vi "Test RoundTrip Nulls.vi"(8 "error in (no error)":errorcluster) -> (0 "error out":errorcluster)   [LabVIEW 2015]
uses:
  <vilib>/Utility/VariantDataType/Type.ctl
  src/Serializer/JSON Serializer/JSON Serializer.lvclass
  src/Deserializer/JSON Deserializer/JSON Deserializer.lvclass
  <vilib>/addons/_JKI Toolkits/Caraya/classes/Test/Test.lvclass
  <vilib>/addons/_JKI Toolkits/Caraya/classes/Assert/Assert.lvclass
  src/JKI JSON Serialization.lvlib
  <vilib>/Utility/VariantDataType/VariantType.lvlib
panel:
  out "Type Enum 2":T1
  out "Wrapped void variant input":cluster{"variant":variant}
  out "Wrapped void variant output":cluster{"variant":variant}
  out "I think this should be {}":string
  out "data":string
  out "Name 3":string
  out "Name":string
  out "output cluster":cluster{"variant container":variant}
  out "I think this should be {\"variant\":null}":string
  out "Type Enum":T1
  out "I think this should be {\"variant\":{}}":string
  out "I think this should be {\"variant\":{}}":string
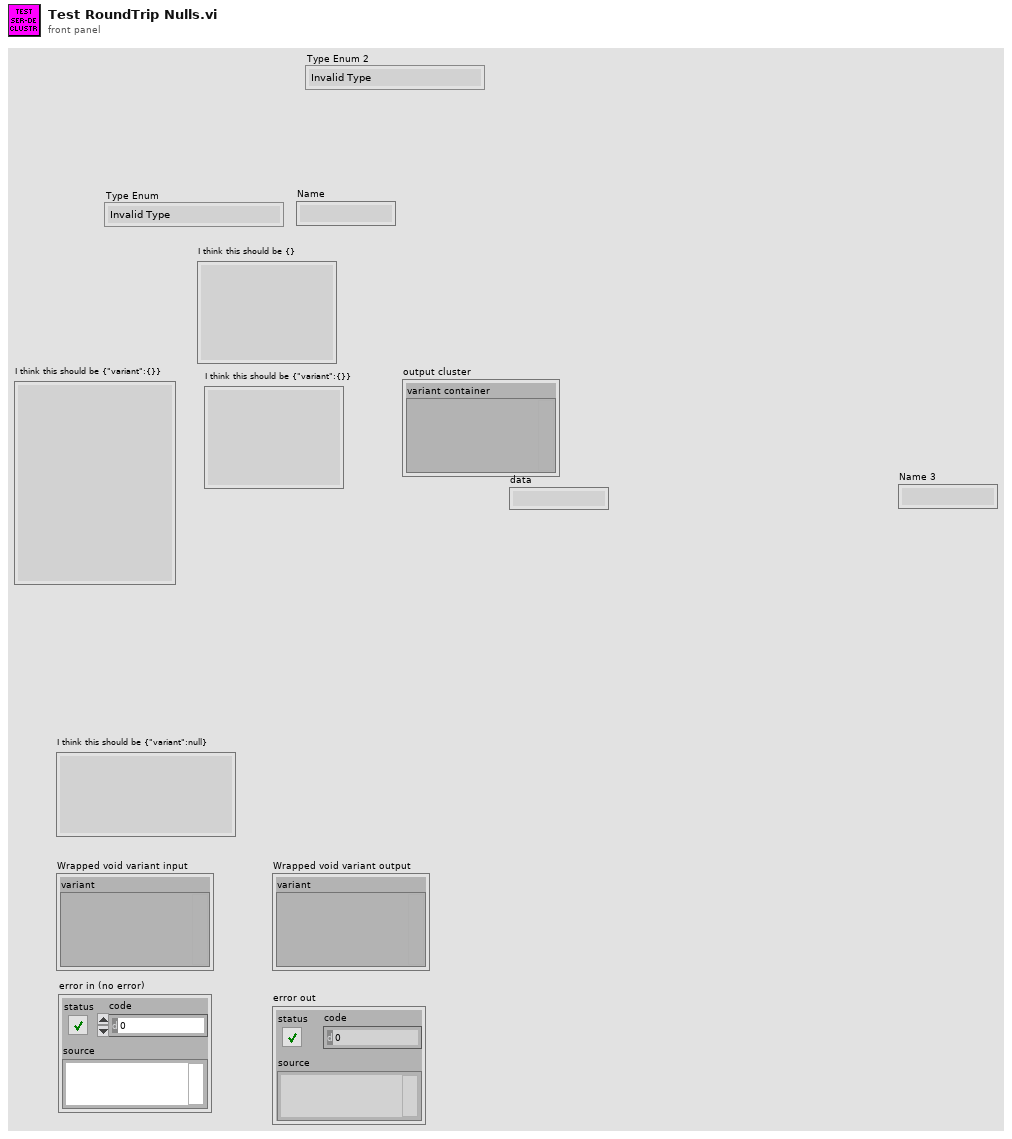
[diagram p1: front panel]
types:
  T1 = typedef "VariantType.lvlib/Type.ctl" = enum8{"Invalid Type", "Void", "I8", "I16", "I32", "I64", "U8", "U16", "U32", "U64", "Single Float", "Double Float", "Extended Float", "Single Complex", "Double Complex", "Extended Complex", "Enum U8", "Enum U16", "Enum U32", "Enum U64", "Single Float With Unit", "Double Float With Unit", "Extended Float With Unit", "Single Complex with Unit", "Double Complex with Unit", "Extended Complex with Unit", "Boolean", "String", "Path", "Picture", "Tag", "Array", "Cluster", "Variant", "LV Variant", "Waveform", "Timestamp", "Digital Waveform", "Digital Data", "ExpressData", "Refnum", "External Data", "VI", "Poly VI", "LabVIEW Class Instance", "Fixed Point"}
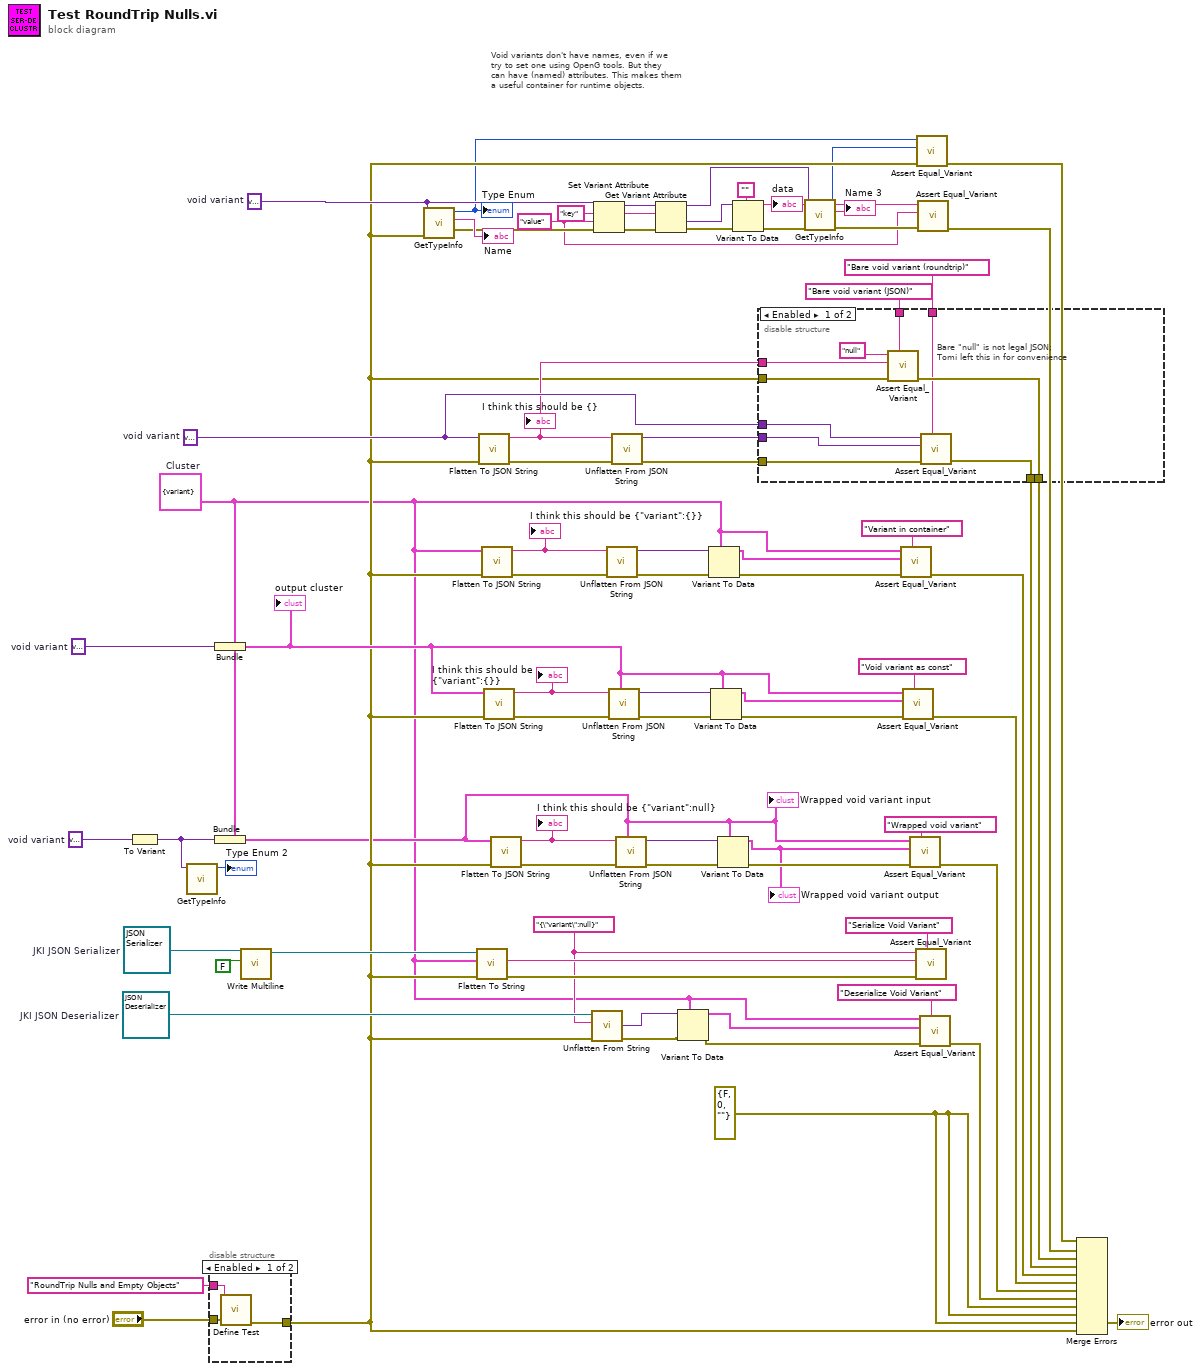
[diagram p0: block diagram]
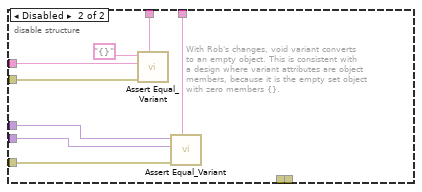
[diagram p2: hidden frame]
diagram:
  w7 = "{\"variant\":null}" ("String")
  w4 = cluster{"variant":variant} {"variant"=variant}  # Cluster
  w13 = "value" ("name")
  w34 = "key" ("name")
  w26 = variant  # void variant
  w39 = variant  # void variant
  w21 = variant  # void variant
  w54 = refnum<class "JSON Deserializer.lvclass"> refnum  # JKI JSON Deserializer
  w57 = refnum<class "JSON Serializer.lvclass"> refnum  # JKI JSON Serializer
  w3 = errorcluster {"status"=FALSE, "code"=0, "source"=""} ("error out")
  w38 = variant  # void variant
  # "Void variants don't have names, even if we\ntry to set one using OpenG tools. But they \ncan have (named) attributes. This makes them\na useful container for runtime objects."
  n1 = To Variant(anything=w39) -> (Variant=w2:variant)
  n2 = call <vilib>:"GetTypeInfo.vi"("Variant"=w2) -> ("Type Enum"=→"Type Enum 2":T1)  [unwired: 6 in, 4 out]
  n3 = disable-structure shown="Enabled" {
    disable-tunnel: "error in (no error)" -> [w81 _]
    disable-tunnel: "RoundTrip Nulls and Empty Objects" ("Label (VI Title)") -> [w80 _]
    disable-tunnel: [w79 _] -> w19
    frame Enabled {
      n4 = call <vilib>:"Define Test.vi"("error in (no error)"=w81, "Label (VI Title)"=w80) -> ("error out"=w79:errorcluster)  [unwired: 9 in]
    }
    frame Disabled {
    }
  }
  n5 = Bundle(cluster=w4, "variant"=w38) -> (w37:cluster{"variant":variant})
  "output cluster" <- w37
  n6 = Bundle(cluster=w4, "variant"=w2) -> (w5:cluster{"variant":variant})
  "Wrapped void variant input" <- w5
  n7 = call-dynamic "Write Multiline.vi"("Multiline"=FALSE, "JSON Serializer in"=w57) -> ("JSON Serializer out"=w78:refnum<class "JSON Serializer.lvclass">)  [unwired: 8 in, 1 out]
  n8 = call <vilib>:"GetTypeInfo.vi"("error in (no error)"=w19, "Variant"=w21) -> ("error out"=w20:errorcluster, "Name"=→"Name":string, "Type Enum"=w11:T1)  [unwired: 5 in, 2 out]
  "Type Enum" <- w11
  n9 = call-dynamic "Flatten To String.vi"("error in (no error)"=w19, "Variant"=w4, "JSON Serializer in"=w78) -> ("error out"=w56:errorcluster, "String"=w8:string)  [unwired: 6 in, 1 out]
  n10 = call "Flatten To JSON String.vi"("error in (no error)"=w19, "Variant"=w26) -> ("error out"=w29:errorcluster, "JSON String"=w25:string)  [unwired: 8 in]
  "I think this should be {}" <- w25
  n11 = call "Flatten To JSON String.vi"("error in (no error)"=w19, "Variant"=w4) -> ("error out"=w62:errorcluster, "JSON String"=w63:string)  [unwired: 8 in]
  "I think this should be {\"variant\":{}}" <- w63
  n12 = call "Flatten To JSON String.vi"("error in (no error)"=w19, "Variant"=w37) -> ("error out"=w73:errorcluster, "JSON String"=w72:string)  [unwired: 8 in]
  "I think this should be {\"variant\":{}}" <- w72
  n13 = call "Flatten To JSON String.vi"("error in (no error)"=w19, "Variant"=w5) -> ("error out"=w41:errorcluster, "JSON String"=w43:string)  [unwired: 8 in]
  "I think this should be {\"variant\":null}" <- w43
  n14 = call-dynamic "Unflatten From String.vi"("error in (no error)"=w19, "String"=w7, "Deserializer in"=w54) -> ("error out"=w50:errorcluster, "Variant"=w52:variant)  [unwired: 6 in, 1 out]
  n15 = Set Variant Attribute(Variant=w21, name=w34, value=w13, error in=w20) -> (Variant out=w35:variant, error out=w18:errorcluster)  [unwired: 1 out]
  n16 = call "Unflatten From JSON String.vi"("error in (no error)"=w62, "JSON String"=w63) -> ("error out"=w66:errorcluster, "Variant"=w64:variant)  [unwired: 8 in]
  n17 = call "Unflatten From JSON String.vi"("Type and Defaults"=w37, "error in (no error)"=w73, "JSON String"=w72) -> ("error out"=w69:errorcluster, "Variant"=w71:variant)  [unwired: 7 in]
  n18 = call "Unflatten From JSON String.vi"("error in (no error)"=w29, "JSON String"=w25) -> ("error out"=w28:errorcluster, "Variant"=w27:variant)  [unwired: 8 in]
  n19 = call "Unflatten From JSON String.vi"("Type and Defaults"=w5, "error in (no error)"=w41, "JSON String"=w43) -> ("error out"=w46:errorcluster, "Variant"=w44:variant)  [unwired: 7 in]
  n20 = Get Variant Attribute(Variant=w35, name=w34, error in=w18) -> (duplicate Variant=w30:variant, value=w32:variant, error out=w17:errorcluster)  [unwired: 1 in, 1 out]
  n21 = Variant To Data(error in=w50, type=w4, Variant=w52) -> (data=w51:cluster{"variant":variant}, error out=w49:errorcluster)
  n22 = Variant To Data(error in=w66, type=w4, Variant=w64) -> (data=w65:cluster{"variant":variant}, error out=w67:errorcluster)
  n23 = Variant To Data(error in=w69, type=w37, Variant=w71) -> (data=w70:cluster{"variant":variant}, error out=w68:errorcluster)
  n24 = Variant To Data(error in=w46, type=w5, Variant=w44) -> (data=w45:cluster{"variant":variant}, error out=w47:errorcluster)
  "Wrapped void variant output" <- w45
  n25 = Variant To Data(error in=w17, type="", Variant=w32) -> (data=w14:string, error out=w16:errorcluster)
  "data" <- w14
  n26 = disable-structure shown="Enabled" {
    disable-tunnel: w28 -> [w91 w99]
    disable-tunnel: w27 -> [w90 w98]
    disable-tunnel: w26 -> [w89 w97]
    disable-tunnel: w25 -> [w88 w96]
    disable-tunnel: w19 -> [w87 w95]
    disable-tunnel: "Bare void variant (JSON)" ("Label") -> [w86 w94]
    disable-tunnel: [w84 _] -> w23
    disable-tunnel: [w83 _] -> w22
    disable-tunnel: "Bare void variant (roundtrip)" ("Label") -> [w82 w92]
    frame Enabled {
      # "Bare \"null\" is not legal JSON;\nTomi left this in for convenience"
      n27 = call <vilib>:"Assert Equal_Variant.vi"("Label"=w86, "error in (no error)"=w87, "Y"=w88, "X"="null" ("JSON String")) -> ("error out"=w83:errorcluster)  [unwired: 7 in]
      n28 = call <vilib>:"Assert Equal_Variant.vi"("Label"=w82, "error in (no error)"=w91, "Y"=w90, "X"=w89) -> ("error out"=w84:errorcluster)  [unwired: 7 in]
    }
    frame Disabled {
      # "With Rob's changes, void variant converts\nto an empty object. This is consistent with\na design where variant attributes are object\nmembers, because it is the empty set object \nwith zero members {}."
      n29 = call <vilib>:"Assert Equal_Variant.vi"("Label"=w94, "error in (no error)"=w95, "Y"=w96, "X"="{}" ("JSON String")) -> ()  [unwired: 7 in, 1 out]
      n30 = call <vilib>:"Assert Equal_Variant.vi"("Label"=w92, "error in (no error)"=w99, "Y"=w98, "X"=w97) -> ()  [unwired: 7 in, 1 out]
    }
  }
  n31 = call <vilib>:"GetTypeInfo.vi"("error in (no error)"=w16, "Variant"=w30) -> ("error out"=w15:errorcluster, "Name"=→"Name 3":string, "Type Enum"=w12:T1)  [unwired: 5 in, 2 out]
  n32 = call <vilib>:"Assert Equal_Variant.vi"("Label"="Variant in container", "error in (no error)"=w67, "Y"=w65, "X"=w4) -> ("error out"=w60:errorcluster)  [unwired: 7 in]
  n33 = call <vilib>:"Assert Equal_Variant.vi"("Label"="Void variant as const", "error in (no error)"=w68, "Y"=w70, "X"=w37) -> ("error out"=w59:errorcluster)  [unwired: 7 in]
  n34 = call <vilib>:"Assert Equal_Variant.vi"("Label"="Wrapped void variant", "error in (no error)"=w47, "Y"=w45, "X"=w5) -> ("error out"=w40:errorcluster)  [unwired: 7 in]
  n35 = call <vilib>:"Assert Equal_Variant.vi"("Label"="Serialize Void Variant", "error in (no error)"=w56, "Y"=w8, "X"=w7) -> ()  [unwired: 7 in, 1 out]
  n36 = call <vilib>:"Assert Equal_Variant.vi"("error in (no error)"=w19, "Y"=w12, "X"=w11) -> ("error out"=w10:errorcluster)  [unwired: 8 in]
  n37 = call <vilib>:"Assert Equal_Variant.vi"("error in (no error)"=w15, "Y"=w13, "X"=w14) -> ("error out"=w9:errorcluster)  [unwired: 8 in]
  n38 = call <vilib>:"Assert Equal_Variant.vi"("Label"="Deserialize Void Variant", "error in (no error)"=w49, "Y"=w51, "X"=w4) -> ("error out"=w48:errorcluster)  [unwired: 7 in]
  n39 = Merge Errors(w10, w9, w22, w23, w60, w59, w40, w48, w3, w3, w3, w19) -> (→"error out":errorcluster)
